vi "NanoStageSetPositions.vi"(7 "error in (no error)":errorcluster, 10 "Config In":T1) -> (0 "error out":errorcluster, 3 "Config Out":T1)   [LabVIEW 2019]
doc: "Generates sample waveforms according to the signal type in the HW Config input."
uses:
  Settings/Settings.ctl
  Support/Hardware Configuration.ctl
  Support/Camera Configuration.ctl
  E:/DevHardSoftware/MMicroscopy/HardwareAdapter/Camera/Dependencies/PVCamNET.dll
  Camera/Dependencies/PVCamNET.dll
  <vilib>/userdefined/High Color/IMAQdx.ctl
  Logging/Logging Configuration.ctl
  controls/UI Configuration.ctl
  Dependencies/Madlib.dll
  Logging/Logging.lvlib
  Settings/Settings.lvlib
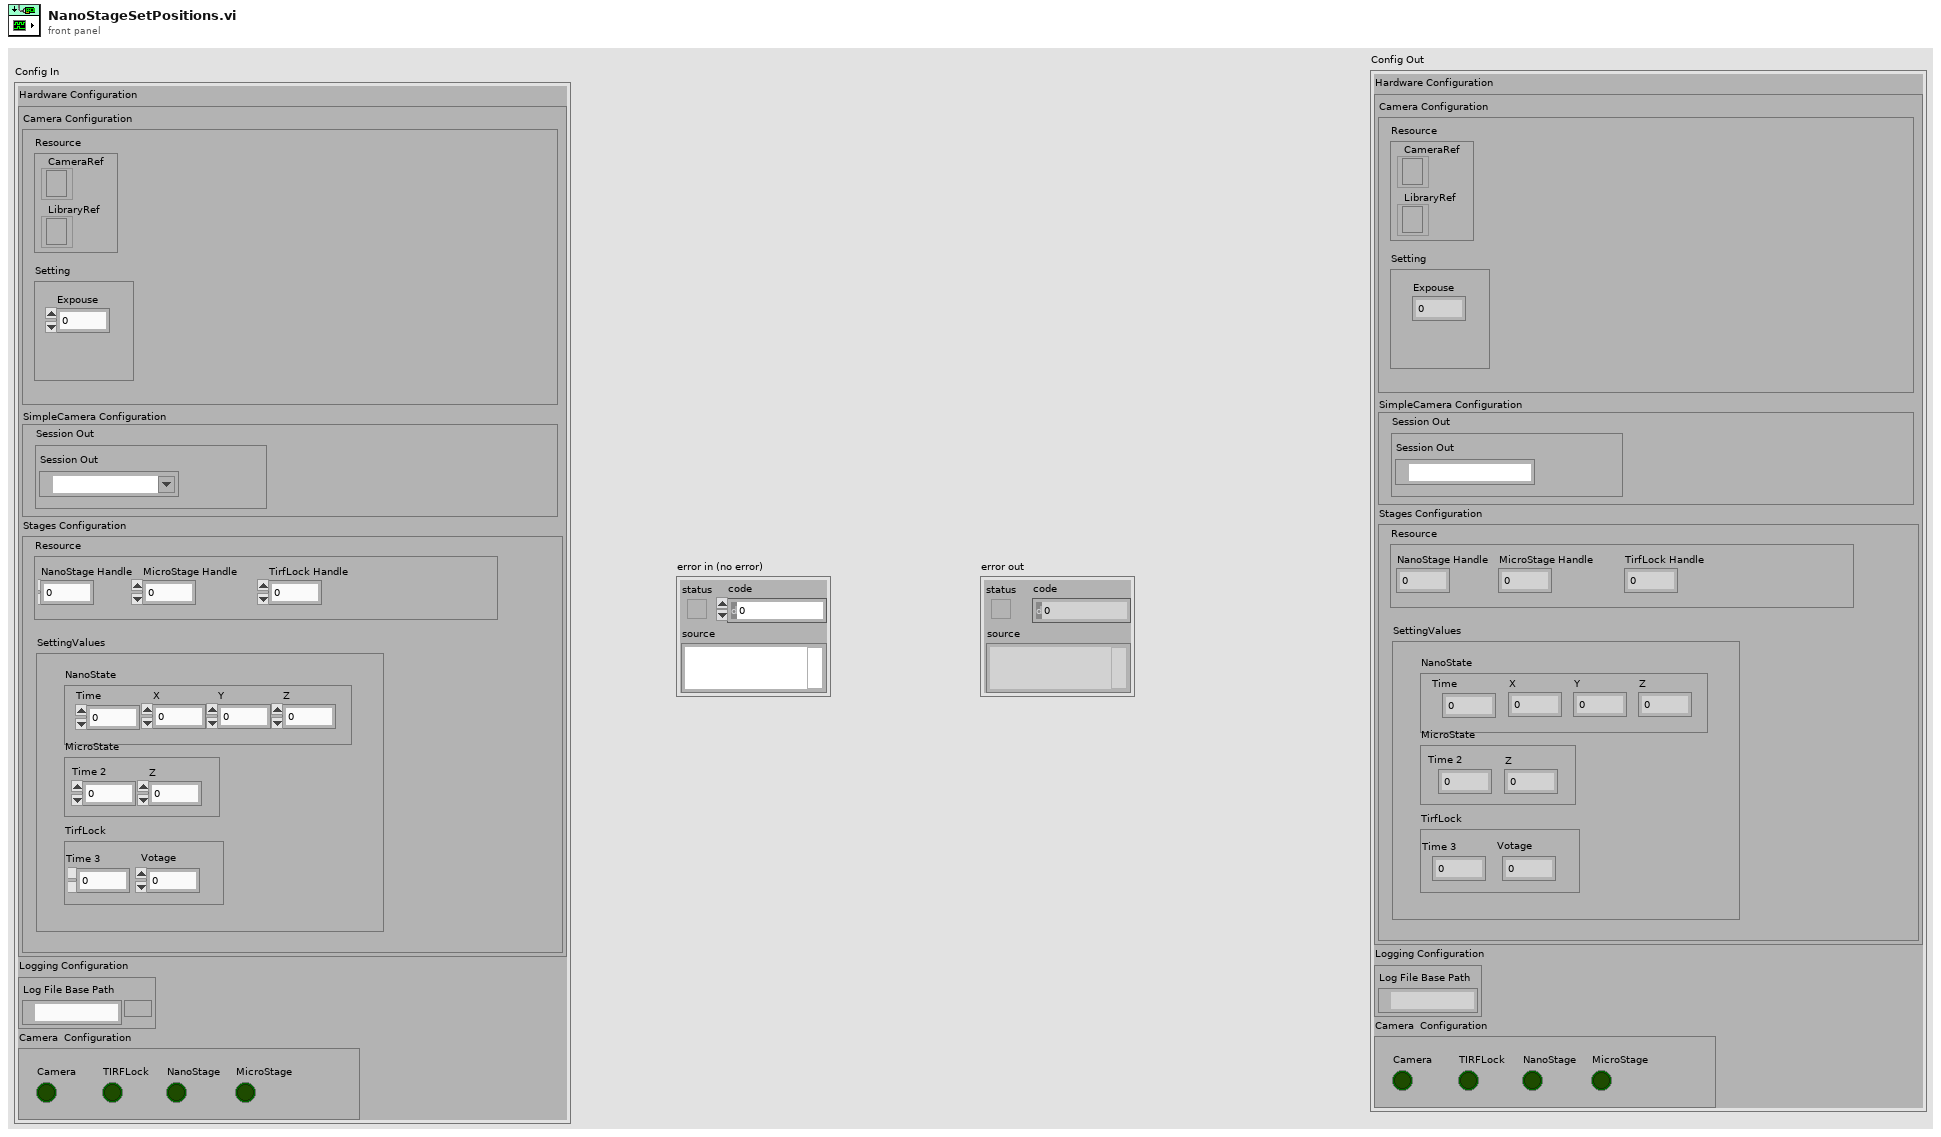
[diagram p1: front panel]
types:
  T1 = typedef "Settings.lvlib/Settings.ctl" = cluster{"Hardware Configuration":T2, "Logging Configuration":T5, "UI Configuration":T6}
  T2 = typedef "Hardware Configuration.ctl" = cluster{"Camera Configuration":T3, "SimpleCamera Configuration":cluster{"Resource":cluster{"Session Out":T4}}, "Stages Configuration":cluster{"Resource":cluster{"NanoStage Handle":i32, "MicroStage Handle":i32, "TirfLock Handle":i32}, "SettingValues":cluster{"NanoState":cluster{"Time":dbl, "X":dbl, "Y":dbl, "Z":dbl}, "MicroState":cluster{"Time 2":dbl, "Z":dbl}, "TirfLock":cluster{"Time 3":dbl, "Votage":dbl}}}}
  T3 = typedef "Camera Configuration.ctl" = cluster{"Resource":cluster{"CameraRef":refnum<k24>, "LibraryRef":refnum<k24>}, "Setting":cluster{"Expouse":dbl}}
  T4 = typedef "IMAQdx.ctl" = refnum<k21>
  T5 = typedef "Logging.lvlib/Logging Configuration.ctl" = cluster{"Log File Base Path":path}
  T6 = typedef "UI Configuration.ctl" = cluster{"Camera":bool, "NanoStage":bool, "MicroStage":bool, "TIRFLock":bool}
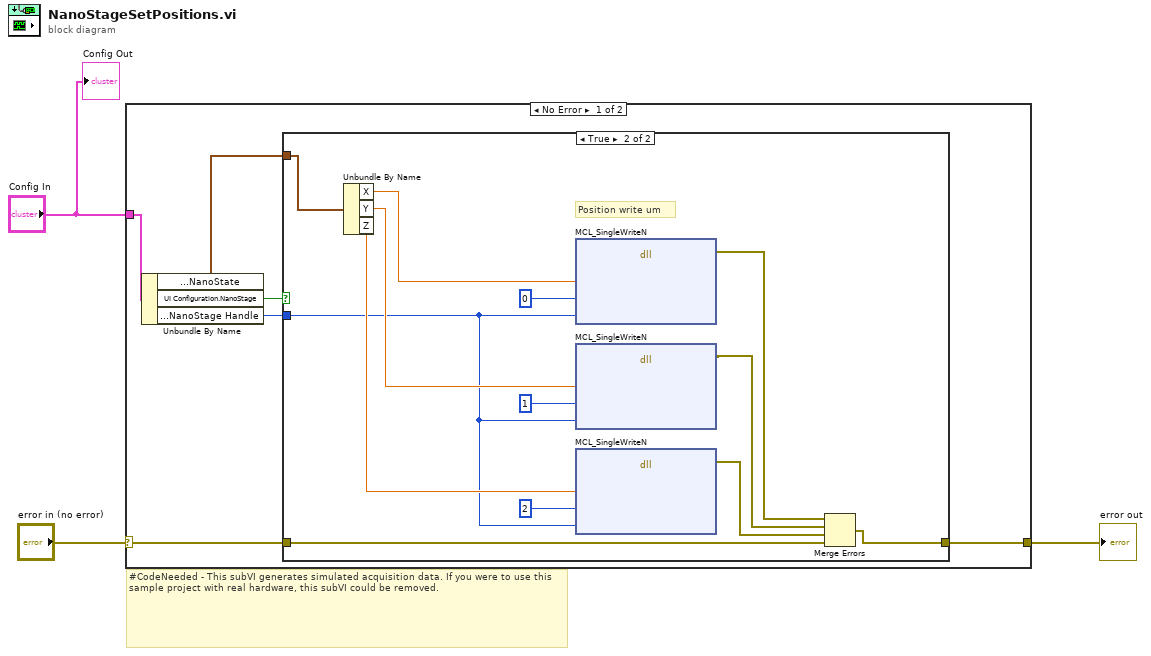
[diagram p0: block diagram]
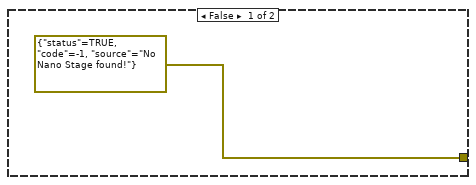
[diagram p2: hidden frame]
diagram:
  # "#CodeNeeded - This subVI generates simulated acquisition data. If you were to use this sample project with real hardware, this subVI could be removed."
  n1 = case shown="No Error" "error in (no error)" {
    selector: "error in (no error)" -> [w7 w24]
    tunnel: [w8 w24] -> w2
    tunnel: "Config In" -> [w4 _]
    frame No Error {
      n2 = Unbundle By Name(w4) -> ("Hardware Configuration.Stages Configuration.SettingValues.NanoState"=w5:cluster{"Time":dbl, "X":dbl, "Y":dbl, "Z":dbl}, "UI Configuration.NanoStage"=w6:bool, "Hardware Configuration.Stages Configuration.Resource.NanoStage Handle"=w9:i32)
      n3 = case shown="True" w6 {
        tunnel: w9 -> [_ w11]
        tunnel: [errorcluster {"status"=TRUE, "code"=-1, "source"="No Nano Stage found!"} ("error IO") w22] -> w8
        tunnel: w7 -> [_ w23]
        tunnel: w5 -> [_ w15]
        frame False {
        }
        frame True {
          # "Position write um"
          n4 = Unbundle By Name(w15) -> ("X"=w14:dbl, "Y"=w13:dbl, "Z"=w12:dbl)
          n5 = dll-call lib="E:/DevHardSoftware/MMicroscopy/HardwareAdapter/Stages/Dependencies/MADLib.dll" fn="MCL_SingleWriteN"("position"=w14, "axis"=u32 0, "handle"=w11) -> (error out=w20:errorcluster)  [unwired: 7 in, 1 out]
          n6 = dll-call lib="E:/DevHardSoftware/MMicroscopy/HardwareAdapter/Stages/Dependencies/Madlib.dll" fn="MCL_SingleWriteN"("position"=w13, "axis"=u32 1, "handle"=w11) -> (error out=w17:errorcluster)  [unwired: 7 in, 1 out]
          n7 = dll-call lib="E:/DevHardSoftware/MMicroscopy/HardwareAdapter/Stages/Dependencies/Madlib.dll" fn="MCL_SingleWriteN"("position"=w12, "axis"=u32 2, "handle"=w11) -> (error out=w16:errorcluster)  [unwired: 7 in, 1 out]
          n8 = Merge Errors(w20, w17, w16, w23) -> (w22:errorcluster)
        }
      }
    }
    frame Error {
    }
  }
  "error out" <- w2
  "Config Out" <- "Config In"
